vi "Encode Parameter in U32.vi"(8 "error in":errorcluster, 9 "parameter definition":T1, 10 "data":dbl, 11 "32-bit word in":u32 format="%032b") -> (0 "error out":errorcluster, 2 "signed?":bool, 3 "32-bit word out":u32 format="%032b")   [LabVIEW 2020, in "32-bit Word.lvclass"]
uses:
  32-bit Word.lvclass
  Parameter Definition.ctl
  <vilib>/NI/NI VeriStand Encoding and Decoding/Encoding.ctl
  4886b350-714d-4ec1-8e20-d9505fba4b81.vi
  fb4e62a2-d19a-48fc-a932-931b706c2fc4.vi
  4886b350-714d-4ec1-8e20-d9505fba4b81.vi/9377bb8f-44b5-4a8f-87f1-966fd5a9edcc.vi
  4886b350-714d-4ec1-8e20-d9505fba4b81.vi/22abf0d2-70bd-4b51-a478-b97a2704f7df.vi
  4886b350-714d-4ec1-8e20-d9505fba4b81.vi/c253b733-33bf-43c6-b07a-ea22f5c7a6f3.vi
  fb4e62a2-d19a-48fc-a932-931b706c2fc4.vi/136dcdcb-2dd3-4a4d-a796-a8f7a3f8e1ac.vi
  fb4e62a2-d19a-48fc-a932-931b706c2fc4.vi/a54b505c-1216-4ef4-8378-3ceda9d188df.vi
  4886b350-714d-4ec1-8e20-d9505fba4b81.vi/22abf0d2-70bd-4b51-a478-b97a2704f7df.vi/9d450a76-0fc9-4555-8e71-4c202274969f.vi
  4886b350-714d-4ec1-8e20-d9505fba4b81.vi/c253b733-33bf-43c6-b07a-ea22f5c7a6f3.vi/9d450a76-0fc9-4555-8e71-4c202274969f.vi
  fb4e62a2-d19a-48fc-a932-931b706c2fc4.vi/a54b505c-1216-4ef4-8378-3ceda9d188df.vi/a7fcce85-1f75-4572-aeaa-ddfd463a7c5f.vi
  <vilib>/NI/NI VeriStand Encoding and Decoding/Encoding and Decoding.lvlib
  ARINC 429.lvclass
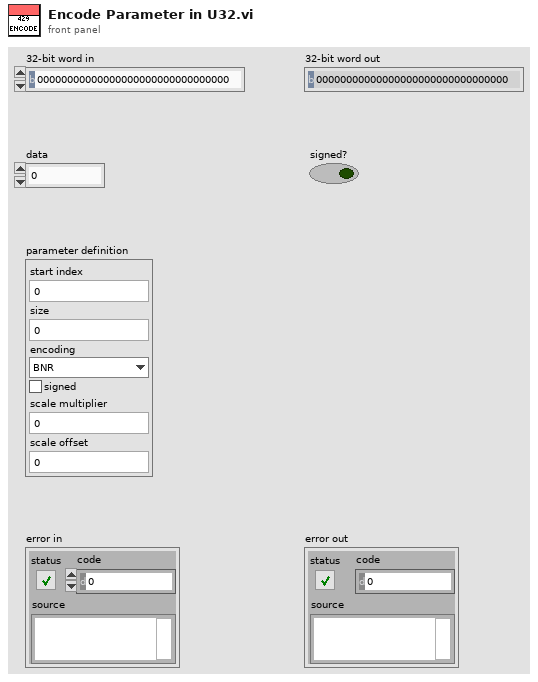
[diagram p1: front panel]
types:
  T1 = typedef "ARINC 429.lvclass/Parameter Definition.ctl" = cluster{"start index":i32, "size":i32, "encoding":T2, "signed":bool, "scale multiplier":dbl, "scale offset":dbl}
  T2 = typedef "Encoding and Decoding.lvlib/Encoding.ctl" = enum16{"BNR", "BCD", "Discrete"}
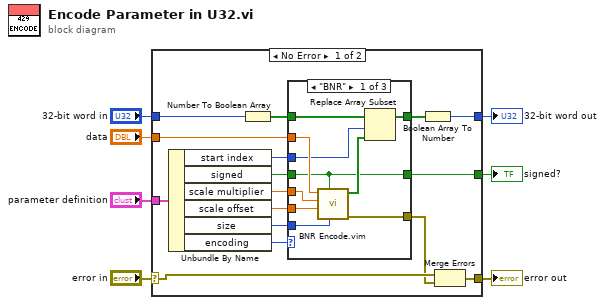
[diagram p0: block diagram]
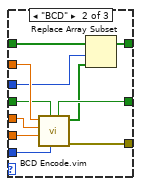
[diagram p2: hidden frame]
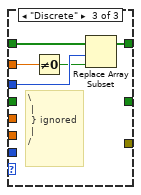
[diagram p3: hidden frame]
diagram:
  n1 = case shown="No Error" "error in" {
    selector: "error in" -> [w9 w51]
    tunnel: [w20 _] -> w7
    tunnel: "parameter definition" -> [w19 _]
    tunnel: "data" -> [w18 _]
    tunnel: [w12 w50] -> w4
    tunnel: "32-bit word in" -> [w11 w50]
    tunnel: [w10 w51] -> w1
    frame No Error {
      n2 = Unbundle By Name(w19) -> ("start index"=w13:i32, "signed"=w14:bool, "scale multiplier"=w17:dbl, "scale offset"=w16:dbl, "size"=w15:i32, "encoding"=w23:T2)
      n3 = Number To Boolean Array(number=w11) -> (Boolean array=w21:bool[])
      n4 = case shown="\"BNR\"" w23 {
        tunnel: w18 -> [w33 w44 w49]
        tunnel: w17 -> [w32 w43 _]
        tunnel: w16 -> [w31 w42 _]
        tunnel: w15 -> [w30 w39 _]
        tunnel: w14 -> [w24 w41 _]
        tunnel: [w24 w40 _] -> w20
        tunnel: [w29 w38 _] -> w8
        tunnel: w13 -> [w27 w36 w48]
        tunnel: w21 -> [w26 w37 w46]
        tunnel: [w25 w34 w45] -> w22
        frame "BNR" {
          n5 = call "BNR Encode.vim"("data size (bits)"=w30, "signed"=w24, "scale offset"=w31, "scale multiplier"=w32, "value"=w33) -> ("error out"=w29:errorcluster, "BNR encoded value"=w28:bool[])  [unwired: 5 in]
          n6 = Replace Array Subset(array=w26, new element=w28, index=w27) -> (w25:bool[])
        }
        frame "BCD" {
          n7 = call "BCD Encode.vim"("data size (bits)"=w39, "signed"=w41, "scale offset"=w42, "scale multiplier"=w43, "value"=w44) -> ("error out"=w38:errorcluster, "BCD encoded value"=w35:bool[], "signed?"=w40:bool)  [unwired: 4 in]
          n8 = Replace Array Subset(array=w37, new element=w35, index=w36) -> (w34:bool[])
        }
        frame "Discrete" {
          # "\\\n |\n } ignored \n |\n/"
          n9 = Not Equal To 0?(x=w49) -> (x != 0?=w47:bool)
          n10 = Replace Array Subset(array=w46, new element=w47, index=w48) -> (w45:bool[])
        }
      }
      n11 = Boolean Array To Number(Boolean array=w22) -> (number=w12:u32)
      n12 = Merge Errors(w9, w8) -> (w10:errorcluster)
    }
    frame Error {
    }
  }
  "error out" <- w1
  "signed?" <- w7
  "32-bit word out" <- w4
